vi "MPM_PowerMonitorType.vi"() -> ()   [LabVIEW 2017]
panel:
  in  "Product_MPM":enum32{"MPM-210/210H", "MPM-220"}(radio) caption="Product"
  in  "MPM_PowerMonitorType":enum16{"DAQ", "MPM_220", "TSL_LOGG"}(ring)
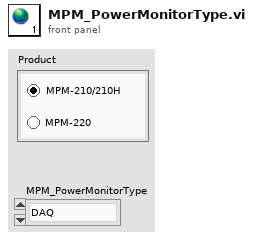
[diagram p1: front panel]
diagram:
